vi "Linear_Comp_Ramp.vi"(2 "Debug Mode":bool, 3 "Elapsed Time (s)":dbl, 4 "State":enum16{"Edit", "Start", "Run", "End", "Idle"}(ring), 5 "Argument List In":string[](array[string])) -> (0 "Status Out":string, 1 "Argument List Out":string[](array[string]))   [LabVIEW 2011]
panel:
  in  "Parameter 3":dbl
  in  "Cancel":bool
  in  "Parameter 1":bool
  in  "Parameter 2":string
  in  "OK":bool
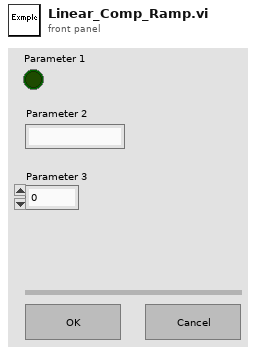
[diagram p1: front panel]
types:
  T1 = enum16{"Discrete", "Continuous", "Instantaneous"}
  T2 = enum32{"Invalid", "Default", "Floating", "Floating/Auto-Hide", "Modal"}
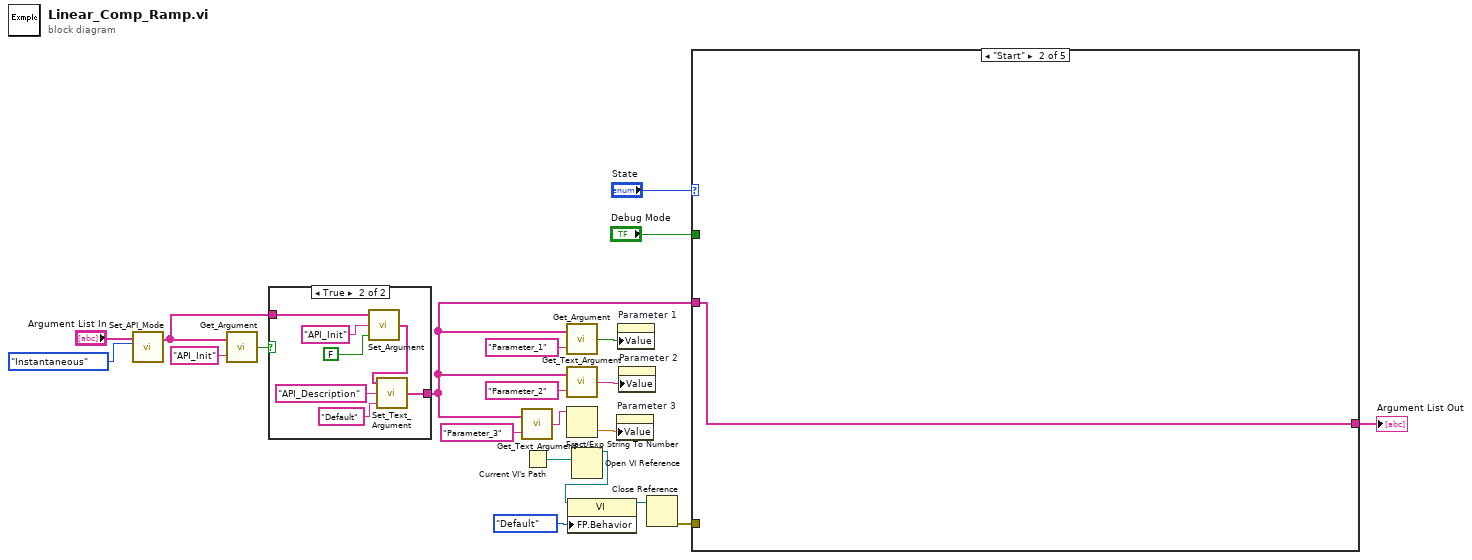
[diagram p0: block diagram]
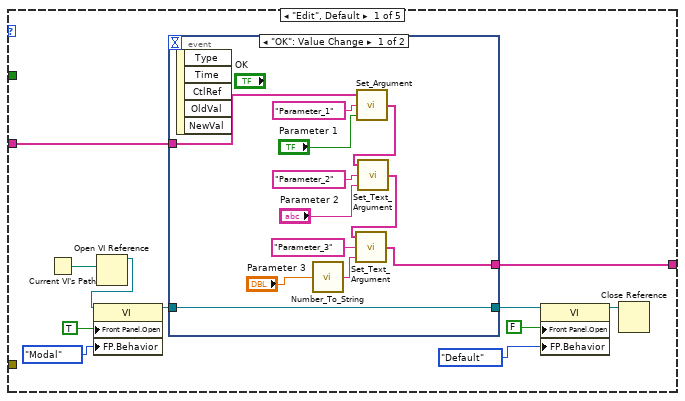
[diagram p3: hidden frame]
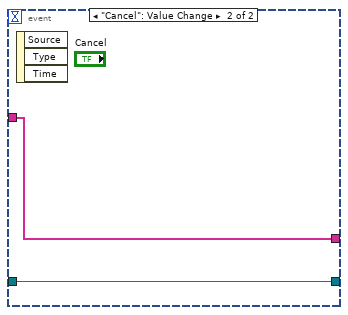
[diagram p4: hidden frame]
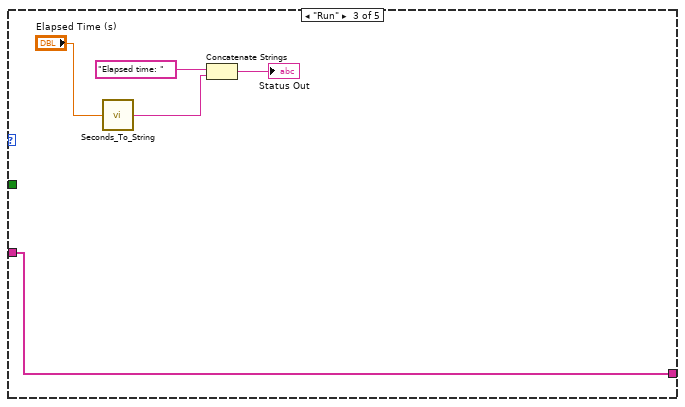
[diagram p5: hidden frame]
diagram:
  n1 = call "Set_API_Mode.vi"("API Mode"=T1."Instantaneous", "Argument List In"="Argument List In") -> ("Argument List Out"=w2:string[])  [unwired: 3 in]
  n2 = call "Get_Argument.vi"("Argument"="API_Init", "Argument List"=w2) -> ("Enabled"=w3:bool)
  n3 = case shown="True" w3 {
    tunnel: w2 -> [w22 w29]
    tunnel: [w22 w24] -> w1
    frame False {
    }
    frame True {
      n4 = call "Set_Argument.vi"("Enable"=FALSE, "Argument"="API_Init", "Argument List In"=w29) -> ("Argument List Out"=w26:string[])
      n5 = call "Set_Text_Argument.vi"("Text"="Default", "Argument"="API_Description", "Argument List In"=w26) -> ("Argument List Out"=w24:string[])
    }
  }
  n6 = call "Get_Text_Argument.vi"("Argument"="Parameter_3", "Argument List"=w1) -> ("Text"=w8:string)
  n7 = Current VI's Path() -> (path=w14:path)
  n8 = call "Get_Argument.vi"("Argument"="Parameter_1", "Argument List"=w1) -> ("Enabled"=w17:bool)
  n9 = call "Get_Text_Argument.vi"("Argument"="Parameter_2", "Argument List"=w1) -> ("Text"=w16:string)
  n10 = Fract/Exp String To Number(string=w8) -> (number=w9:dbl)  [unwired: 4 out]
  n11 = Open VI Reference(vi path=w14) -> (vi reference=w13:refnum<vi>)  [unwired: 1 in, 5 out]
  n12 = property class="VI"(reference=w13, "FP.Behavior"=T2."Default" ("Front Panel Window:Behavior")) -> (reference out=w11:refnum<vi>)  [unwired: 1 in, 1 out]
  n13 = property on="Parameter 3" class="DigNum (strict)"("Value"=w9) -> ()  [unwired: 2 in, 2 out]
  n14 = property on="Parameter 1" class="Bool (strict)"("Value"=w17) -> ()  [unwired: 2 in, 2 out]
  n15 = property on="Parameter 2" class="Str"("Value"=w16) -> ()  [unwired: 2 in, 2 out]
  n16 = Close Reference(reference=w11) -> (error out=w10:errorcluster)  [unwired: 1 in]
  n17 = case shown="\"Start\"" "State" {
    tunnel: [w40 w55 w56 w61 w62] -> w20
    tunnel: w1 -> [w39 w55 w56 w61 w62]
    tunnel: "Debug Mode" -> [_ _ _ _ _]
    tunnel: w10 -> [_ _ _ _ _]
    frame "Edit", Default {
      n18 = Current VI's Path() -> (path=w34:path)
      n19 = Open VI Reference(vi path=w34) -> (vi reference=w33:refnum<vi>)  [unwired: 1 in, 5 out]
      n20 = property class="VI"(reference=w33, "Front Panel.Open"=TRUE ("Front Panel Window:Open"), "FP.Behavior"=T2."Modal" ("Front Panel Window:Behavior")) -> (reference out=w37:refnum<vi>)  [unwired: 1 in, 1 out]
      n21 = event shown="[0] \"OK\": Value Change" {
        selector: _ -> [_ _]
        dyn-events: _ -> [_ _]
        timeout: _ -> [_ _]
        tunnel: w39 -> [w48 w53]
        tunnel: [w43 w53] -> w40
        tunnel: [w46 w54] -> w36
        tunnel: w37 -> [w46 w54]
        event "OK": Value Change {
          n22 = event-data() -> ()  [unwired: 6 out]
          n23 = call "Number_To_String.vi"("Number"="Parameter 3") -> ("String"=w42:string)
          n24 = call "Set_Argument.vi"("Enable"="Parameter 1", "Argument"="Parameter_1", "Argument List In"=w48) -> ("Argument List Out"=w47:string[])
          n25 = call "Set_Text_Argument.vi"("Text"="Parameter 2", "Argument"="Parameter_2" ("Text"), "Argument List In"=w47) -> ("Argument List Out"=w44:string[])
          n26 = call "Set_Text_Argument.vi"("Text"=w42, "Argument"="Parameter_3", "Argument List In"=w44) -> ("Argument List Out"=w43:string[])
        }
        event "Cancel": Value Change {
          n27 = event-data() -> ()  [unwired: 4 out]
        }
      }
      n28 = property class="VI"(reference=w36, "Front Panel.Open"=FALSE ("Front Panel Window:Open"), "FP.Behavior"=T2."Default" ("Front Panel Window:Behavior")) -> (reference out=w30:refnum<vi>)  [unwired: 1 in, 1 out]
      n29 = Close Reference(reference=w30) -> ()  [unwired: 1 in, 1 out]
    }
    frame "Start" {
    }
    frame "Run" {
      n30 = call "Seconds_To_String.vi"("Seconds"="Elapsed Time (s)") -> ("Output String"=w58:string)
      n31 = Concatenate Strings("Elapsed time: " ("string"), w58) -> (→"Status Out":string)
    }
    frame "End" {
    }
    frame "Idle" {
    }
  }
  "Argument List Out" <- w20
